vi "BasicTest.vi"() -> ()   [LabVIEW 2014]
panel:
  in  "Yaw":sgl(slide) scale=-180.0..180.0
  out "data In":string
  out "Boolean":bool
  in  "Override\nplanepath":bool
  in  "Roll":sgl(slide) scale=-180.0..180.0
  in  "Pitch":sgl(slide) scale=-90.0..90.0
  out "data out":string
  in  "stop":bool
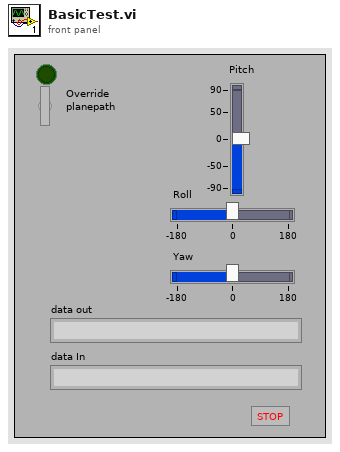
[diagram p1: front panel]
types:
  T1 = cluster{"[0]":sgl, "[1]":sgl, "[2]":sgl, "[3]":sgl}
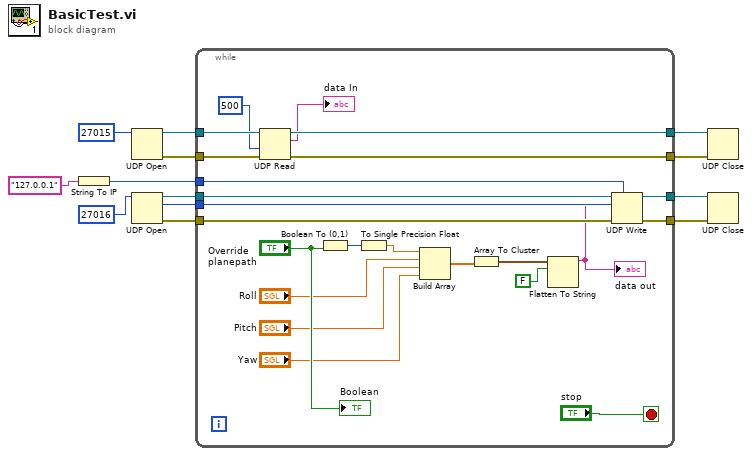
[diagram p0: block diagram]
diagram:
  n1 = String To IP(1:"127.0.0.1" ("name")) -> (0:w3:u32)
  n2 = UDP Open(11:u16 27015 ("port")) -> (port=w11:refnum<k16>, 0:w13:errorcluster)  [unwired: 4 in, 1 out]
  n3 = UDP Open(11:u16 27016 ("port")) -> (port=w7:refnum<k16>, 0:w8:errorcluster, 2:w1:u16)  [unwired: 4 in]
  n4 = while {
    tunnel: w13 -> [w36]
    tunnel: [w35] -> w12
    tunnel: w11 -> [w34]
    tunnel: [w33] -> w10
    tunnel: w8 -> [w30]
    tunnel: w7 -> [w29]
    tunnel: [w28] -> w6
    tunnel: [w27] -> w5
    tunnel: w3 -> [w26]
    tunnel: w1 -> [w25]
    stop <- "stop" stop-if-true
    n5 = UDP Read(connection ID=w34, timeout ms (25000)=500, 8:w36) -> (data out=→"data In":string, error out=w35:errorcluster, 3:w33:refnum<k16>)  [unwired: 1 in, 2 out]
    n6 = Boolean To (0,1)(Boolean="Override\nplanepath") -> (0, 1=w21:i16)
    n7 = To Single Precision Float(number=w21) -> (single precision float=w20:sgl)
    n8 = Build Array(w20, "Roll", "Pitch", "Yaw") -> (w24:sgl[])
    n9 = Array To Cluster(array=w24) -> (cluster=w23:T1)
    n10 = Flatten To String(anything=w23, prepend array or string size? (T)=FALSE) -> (data string=w18:string)  [unwired: 2 in, 2 out]
    "data out" <- w18
    n11 = UDP Write(address=w26, port or service name=w25, connection ID=w29, data in=w18, 8:w30) -> (error out=w28:errorcluster, 3:w27:refnum<k16>)  [unwired: 1 in]
    "Boolean" <- "Override\nplanepath"
  }
  n12 = UDP Close(connection ID=w10, 8:w12) -> ()  [unwired: 2 out]
  n13 = UDP Close(connection ID=w5, 8:w6) -> ()  [unwired: 2 out]
